vi "MoveWrist.vi"() -> ()   [LabVIEW 2018]
uses:
  Framework/Robot Global Data.vi
panel:
  in  "Down":bool
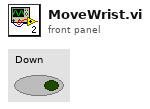
[diagram p1: front panel]
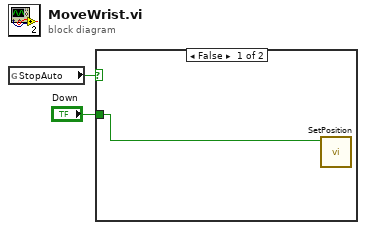
[diagram p0: block diagram]
diagram:
  n1 = global read "Robot Global Data.vi" "StopAuto"() -> (w2:bool)
  n2 = case shown="False" w2 {
    tunnel: "Down" -> [w3 _]
    frame False {
      n3 = call "SetPosition.vi"("Down and out?"=w3) -> ()  [unwired: 10 in, 1 out]
    }
    frame True {
    }
  }
